vi "Do.vi"(8 "error in":errorcluster, 10 "Actor in":refnum<class "Actor.lvclass">, 11 "Change O3 Lamp Run MSG":refnum<class "Change O3 Lamp Run MSG.lvclass">) -> (0 "error out":errorcluster, 2 "Actor out":refnum<class "Actor.lvclass">)   [LabVIEW 2014, in "Calibration.lvlib" / "Change O3 Lamp Run MSG.lvclass"]
doc: "(<B>Filename</B>: Actor Framework.lvlib:Message.lvclass:Do.vi)\n\nDefines what a message does when it is received by an actor. Generally, a message instructs an actor to invoke one of its methods. By default, this method does nothing. A child class must override it to define behavior. Create a child class by using the Actor Framework Message Maker dialog box."
uses:
  Change O3 Lamp Run MSG.lvclass
  <vilib>/ActorFramework/Actor/Actor.lvclass
  Change O3 Lamp Run MSG.lvclass/Change O3 Lamp Run MSG.ctl
  O3 Frequency Train Actor.lvclass
  SuperActor/SuperClass.lvclass/SuperClass.ctl
  O3 Frequency Train Actor.lvclass/O3 Frequency Train Actor.ctl
  SuperActor/Read Log Session.vi
  Accessors/Read RunNotifier.vi
  <userlib>/_Session Fwk/Session - Root.lvclass
  reusable/Session APIs/Session Log/System Log.lvclass
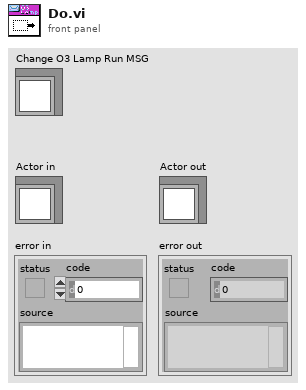
[diagram p1: front panel]
types:
  T1 = typedef "Session - Root.lvclass/Session Handle.ctl" = refnum<data-value>
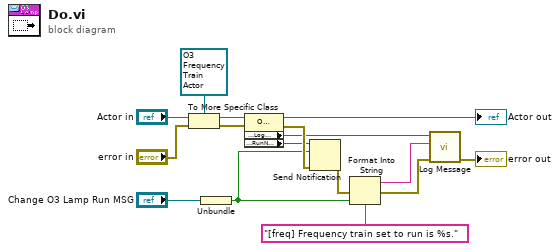
[diagram p0: block diagram]
diagram:
  n1 = To More Specific Class(target class=refnum<class "O3 Frequency Train Actor.lvclass"> refnum ("Calibration.lvlib:O3 Frequency Train Actor.lvclass"), reference="Actor in", error in="error in") -> (specific class reference=w14:refnum<class "O3 Frequency Train Actor.lvclass">, error out=w10:errorcluster)
  n2 = Unbundle("Change O3 Lamp Run MSG") -> (w7:bool)
  n3 = property class="O3 Frequency Train Actors"(reference=w14, error in=w10) -> (reference out=→"Actor out":refnum<class "O3 Frequency Train Actor.lvclass">, error out=w9:errorcluster, "Accessors:Log Session"=w2:T1, "Accessors:RunNotifier"=w1:refnum<notifier>)
  n4 = Send Notification(notification=w7, notifier=w1, error in (no error)=w9) -> (error out=w6:errorcluster)  [unwired: 1 out]
  n5 = Format Into String(format string="[freq] Frequency train set to run is %s.", error in=w6, w7) -> (resulting string=w3:string, error out=w5:errorcluster)  [unwired: 1 in]
  n6 = call "Log Message.vi"("error in"=w5, "MSG In"=w3, "session in"=w2) -> ("error out"=→"error out":errorcluster)  [unwired: 7 in, 1 out]
